vi "DS1000Z_Image_Grabber.vi"() -> ()   [LabVIEW 2020]
uses:
  <vilib>/Instr/_visa.llb/VISA Find Search Mode.ctl
  <vilib>/Utility/error.llb/DialogType.ctl
  <vilib>/Platform/browser.llb/Open URL in Default Browser (string).vi
  rigol_ds1000_series/RIGOL DS1000 Series/RIGOL DS1000 Series.lvlib
panel:
  in  "weblink":bool
  in  "Mode":u16(ring) items=["Single", "Stop"]
  in  "Set Trigger":bool
  in  "Trigger Delay":u32 format="%d sec"
  in  "Get Image":bool
  in  "Capture Delay":u32 format="%d sec"
  in  "File Name":string
  in  "Capture Storage Location":path
  in  "Invert":bool
  in  "Device Location":string(combo)
  in  "Format":u16(ring)=2 items=["24b BMP", "8b BMP", "PNG", "JPEG", "TIFF"]
  in  "Colour?":u16(ring) items=["Colour", "Grayscale"]
  # "Rigol DS1000Z-Series Oscilloscope PC Interface"
  # "© 2020 NixLabs  Version 0.56"
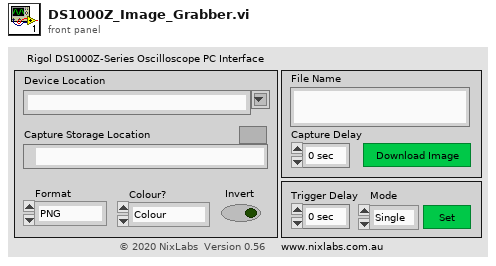
[diagram p1: front panel]
types:
  T1 = enum8{"Enabled", "Disabled", "Disabled and Grayed Out"}
  T2 = typedef "VISA Find Search Mode.ctl" = u32
  T3 = enum16{"big-endian, network order", "native, host order", "little-endian"}
  T4 = typedef "DialogType.ctl" = u16
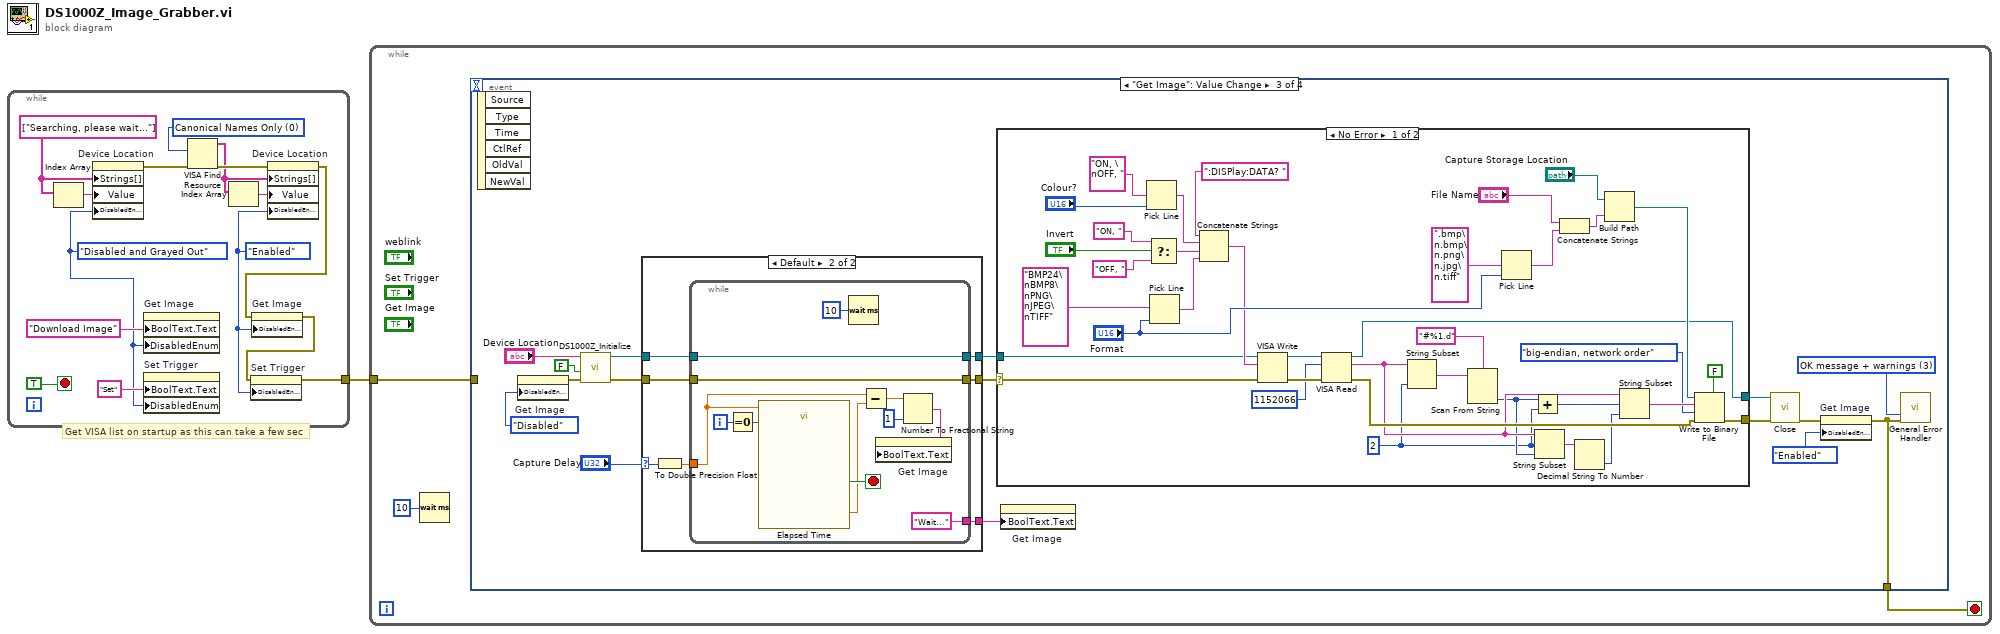
[diagram p0: block diagram]
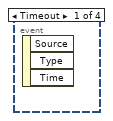
[diagram p2: hidden frame]
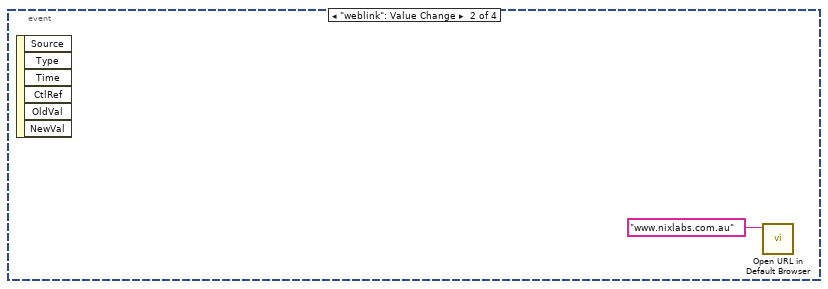
[diagram p3: hidden frame]
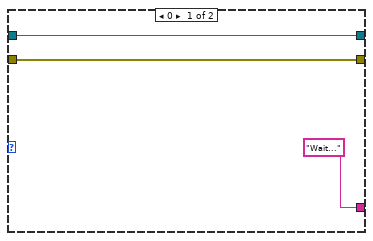
[diagram p4: hidden frame]
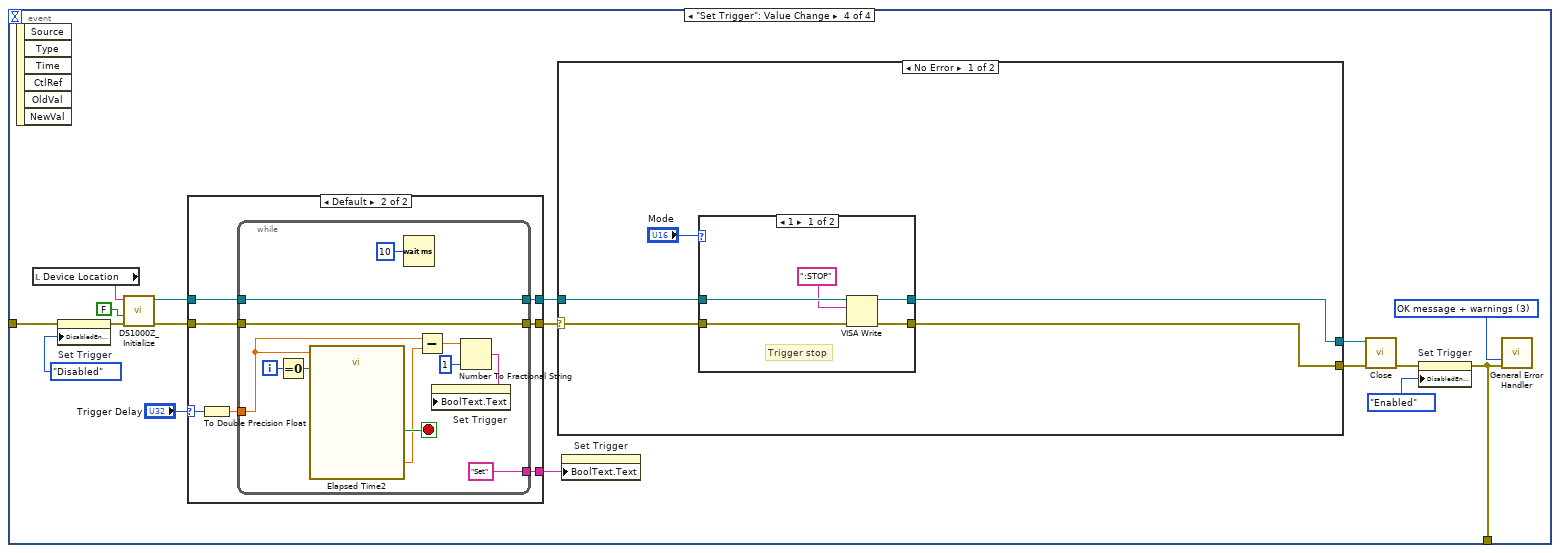
[diagram p6: hidden frame]
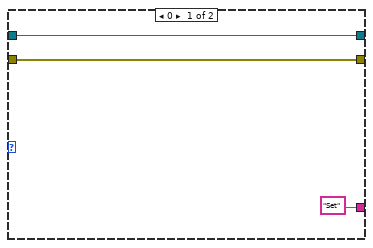
[diagram p7: hidden frame]
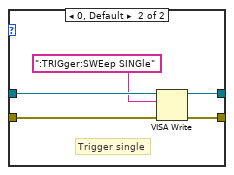
[diagram p8: hidden frame]
diagram:
  # "Get VISA list on startup as this can take a few sec"
  n1 = while {
    tunnel: [w2] -> w1
    stop <- TRUE stop-if-true
    w5 = T1."Enabled" ("Disabled")
    w6 = T1."Disabled and Grayed Out" ("Disabled")
    w10 = string[] ["Searching, please wait..."] ("array")
    w16 = T2 0 items=["Canonical Names Only"=0, "Aliases Only"=2, "Include Matching Aliases"=3, "Include All Aliases"=4] ("Search Mode")
    n2 = Index Array(array=w10) -> (element=w11:string)  [unwired: 1 in]
    n3 = property on="Device Location" class="CmbBox"("Strings[]"=w10, "Value"=w11, "DisabledEnum"=w6) -> (error out=w12:errorcluster)  [unwired: 2 in, 1 out]
    n4 = property on="Get Image" class="Bool"("BoolText.Text"="Download Image" ("Boolean Text.Text"), "DisabledEnum"=w6) -> ()  [unwired: 2 in, 2 out]
    n5 = property on="Set Trigger" class="Bool"("BoolText.Text"="Set" ("Boolean Text.Text"), "DisabledEnum"=w6) -> ()  [unwired: 2 in, 2 out]
    n6 = VISA Find Resource(8:w12, 10:w16) -> (0:w15:errorcluster, 3:w14:string[])  [unwired: 1 in, 1 out]
    n7 = Index Array(array=w14) -> (element=w13:string)  [unwired: 1 in]
    n8 = property on="Device Location" class="CmbBox"(error in=w15, "Strings[]"=w14, "Value"=w13, "DisabledEnum"=w5) -> (error out=w4:errorcluster)  [unwired: 1 in, 1 out]
    n9 = property on="Get Image" class="Bool"(error in=w4, "DisabledEnum"=w5) -> (error out=w3:errorcluster)  [unwired: 1 in, 1 out]
    n10 = property on="Set Trigger" class="Bool"(error in=w3, "DisabledEnum"=w5) -> (error out=w2:errorcluster)  [unwired: 1 in, 1 out]
  }
  n11 = while {
    tunnel: w1 -> [w17]
    stop <- w19 stop-if-true
    n12 = Wait (ms)(milliseconds to wait=u32 10) -> ()  [unwired: 1 out]
    n13 = event shown="[2] \"Get Image\": Value Change" {
      selector: _ -> [_ _ _ _]
      dyn-events: _ -> [_ _ _ _]
      timeout: _ -> [_ _ _ _]
      tunnel: [_ _ w22 w101] -> w19
      tunnel: w17 -> [_ _ _ w99]
      event Timeout {
        n14 = event-data() -> ()  [unwired: 1 in, 3 out]
      }
      event "weblink": Value Change {
        n15 = event-data() -> ()  [unwired: 1 in, 6 out]
        n16 = call-poly <vilib>:"Open URL in Default Browser.vi"("URL"="www.nixlabs.com.au") -> ()  [unwired: 5 in, 2 out]
      }
      event "Get Image": Value Change {
        w36 = T4 3 items=["no dialog", "OK message", "continue or stop message", "OK message + warnings", "continue/stop + warnings"] ("type of dialog (OK msg:1)")
        n17 = event-data() -> ()  [unwired: 1 in, 6 out]
        n18 = property on="Get Image" class="Bool"("DisabledEnum"=T1."Disabled" ("Disabled")) -> (error out=w25:errorcluster)  [unwired: 2 in, 1 out]
        n19 = call "DS1000Z_Initialize.vi"("error in (no error)"=w25, "Reset (True)"=FALSE, "VISA resource name"="Device Location") -> ("error out"=w30:errorcluster, "VISA resource name out"=w32:refnum<visa-resource-name>)  [unwired: 7 in]
        n20 = case shown="Default" "Capture Delay" {
          selector: "Capture Delay" -> [_ w41]
          tunnel: [w38 w46] -> w33
          tunnel: w32 -> [w38 w45]
          tunnel: [w39 w44] -> w31
          tunnel: w30 -> [w39 w43]
          tunnel: ["Wait..." w42] -> w29
          frame 0 {
          }
          frame Default {
            n21 = To Double Precision Float(number=w41) -> (double precision float=w40:dbl)
            n22 = while {
              tunnel: [w56] -> w46
              tunnel: w45 -> [w56]
              tunnel: [w55] -> w44
              tunnel: w43 -> [w55]
              tunnel: ["Wait..."] -> w42
              tunnel: w40 -> [w52]
              i -> [w48]
              stop <- w53 stop-if-true
              n23 = Equal To 0?(x=w48) -> (x = 0?=w47:bool)
              n24 = call "Elapsed Time"("Time Target (s)"=w52, "Reset"=w47) -> ("Elapsed Time (s)"=w51:dbl, "Time has Elapsed"=w53:bool)  [unwired: 10 in, 6 out]
              n25 = Wait (ms)(milliseconds to wait=u32 10) -> ()  [unwired: 1 out]
              n26 = Subtract(x=w52, y=w51) -> (x-y=w50:dbl)
              n27 = Number To Fractional String(number=w50, precision (6)=i16 1) -> (F-format string=w57:string)  [unwired: 2 in]
              n28 = property on="Get Image" class="Bool"("BoolText.Text"=w57) -> ()  [unwired: 2 in, 2 out]
            }
          }
        }
        n29 = case shown="No Error" w31 {
          selector: w31 -> [w60 w97]
          tunnel: [w95 w97] -> w35
          tunnel: w33 -> [w59 w96]
          tunnel: [w61 w96] -> w34
          frame No Error {
            w64 = 2 ("length (rest)")
            n30 = Pick Line(multi-line string="ON, \nOFF, ", line index="Colour?") -> (output string=w83:string)  [unwired: 1 in]
            n31 = Select(t="ON, " ("write buffer"), s="Invert", f="OFF, " ("write buffer")) -> (s? t:f=w84:string)
            n32 = Pick Line(multi-line string="BMP24\nBMP8\nPNG\nJPEG\nTIFF", line index="Format") -> (output string=w85:string)  [unwired: 1 in]
            n33 = Concatenate Strings(":DISPlay:DATA? " ("write buffer"), w83, w84, w85) -> (w86:string)
            n34 = VISA Write(VISA resource name=w59, write buffer=w86, error in (no error)=w60) -> (VISA resource name out=w74:refnum<visa-resource-name>, error out=w73:errorcluster)  [unwired: 1 out]
            n35 = VISA Read(VISA resource name=w74, byte count=u32 1152066, error in (no error)=w73) -> (VISA resource name out=w61:refnum<visa-resource-name>, read buffer=w81:string, error out=w82:errorcluster)  [unwired: 1 out]
            n36 = String Subset(string=w81, length (rest)=w64) -> (substring=w75:string)  [unwired: 1 in]
            n37 = Scan From String(format string="#%1.d", input string=w75) -> (output 1=w77:i32)  [unwired: 3 in, 3 out]
            n38 = Pick Line(multi-line string=".bmp\n.bmp\n.png\n.jpg\n.tiff", line index="Format") -> (output string=w89:string)  [unwired: 1 in]
            n39 = Add(x=w77, y=w64) -> (x+y=w79:i32)
            n40 = String Subset(string=w81, offset (0)=w64, length (rest)=w77) -> (substring=w76:string)
            n41 = Concatenate Strings("File Name", w89) -> (w88:string)
            n42 = Decimal String To Number(string=w76) -> (number=w78:i32)  [unwired: 2 in, 1 out]
            n43 = Build Path(base path="Capture Storage Location", name or relative path=w88) -> (appended path=w87:path)
            n44 = String Subset(string=w81, offset (0)=w79, length (rest)=w78) -> (substring=w80:string)
            n45 = Write to Binary File(file (use dialog)=w87, data=w80, error in=w82, 5:FALSE ("prepend array or string size? (T)"), 9:T3."big-endian, network order" ("byte order (0:big-endian, network order)")) -> (error out=w95:errorcluster)  [unwired: 1 in, 2 out]
          }
          frame Error {
          }
        }
        n46 = property on="Get Image" class="Bool"("BoolText.Text"=w29) -> ()  [unwired: 2 in, 2 out]
        n47 = call "Close.vi"("error in (no error)"=w35, "VISA resource name"=w34) -> ("error out"=w23:errorcluster)  [unwired: 9 in]
        n48 = property on="Get Image" class="Bool"(error in=w23, "DisabledEnum"=T1."Enabled" ("Disabled")) -> (error out=w22:errorcluster)  [unwired: 1 in, 1 out]
        n49 = call <vilib>:"General Error Handler.vi"("type of dialog (OK msg:1)"=w36, "error in (no error)"=w22) -> ()  [unwired: 9 in, 5 out]
      }
      event "Set Trigger": Value Change {
        w114 = T4 3 items=["no dialog", "OK message", "continue or stop message", "OK message + warnings", "continue/stop + warnings"] ("type of dialog (OK msg:1)")
        n50 = event-data() -> ()  [unwired: 1 in, 6 out]
        n51 = local read "Device Location"() -> (w98:string)
        n52 = property on="Set Trigger" class="Bool"(error in=w99, "DisabledEnum"=T1."Disabled" ("Disabled")) -> (error out=w104:errorcluster)  [unwired: 1 in, 1 out]
        n53 = call "DS1000Z_Initialize.vi"("error in (no error)"=w104, "Reset (True)"=FALSE, "VISA resource name"=w98) -> ("error out"=w108:errorcluster, "VISA resource name out"=w110:refnum<visa-resource-name>)  [unwired: 7 in]
        n54 = case shown="Default" "Trigger Delay" {
          selector: "Trigger Delay" -> [_ w119]
          tunnel: [w116 w124] -> w111
          tunnel: w110 -> [w116 w123]
          tunnel: [w117 w122] -> w109
          tunnel: w108 -> [w117 w121]
          tunnel: ["Set" w120] -> w107
          frame 0 {
          }
          frame Default {
            n55 = To Double Precision Float(number=w119) -> (double precision float=w118:dbl)
            n56 = while {
              tunnel: [w134] -> w124
              tunnel: w123 -> [w134]
              tunnel: [w133] -> w122
              tunnel: w121 -> [w133]
              tunnel: ["Set"] -> w120
              tunnel: w118 -> [w130]
              i -> [w126]
              stop <- w131 stop-if-true
              n57 = Equal To 0?(x=w126) -> (x = 0?=w125:bool)
              n58 = call "Elapsed Time2"("Time Target (s)"=w130, "Reset"=w125) -> ("Elapsed Time (s)"=w129:dbl, "Time has Elapsed"=w131:bool)  [unwired: 10 in, 6 out]
              n59 = Wait (ms)(milliseconds to wait=u32 10) -> ()  [unwired: 1 out]
              n60 = Subtract(x=w130, y=w129) -> (x-y=w128:dbl)
              n61 = Number To Fractional String(number=w128, precision (6)=i16 1) -> (F-format string=w135:string)  [unwired: 2 in]
              n62 = property on="Set Trigger" class="Bool"("BoolText.Text"=w135) -> ()  [unwired: 2 in, 2 out]
            }
          }
        }
        n63 = case shown="No Error" w109 {
          selector: w109 -> [w141 w153]
          tunnel: [w137 w153] -> w113
          tunnel: w111 -> [w140 w152]
          tunnel: [w139 w152] -> w112
          frame No Error {
            n64 = case shown="1" "Mode" {
              tunnel: w141 -> [w146 w151]
              tunnel: w140 -> [w145 w150]
              tunnel: [w143 w148] -> w139
              tunnel: [w142 w147] -> w137
              frame 1 {
                # "Trigger stop"
                n65 = VISA Write(VISA resource name=w145, write buffer=":STOP", error in (no error)=w146) -> (VISA resource name out=w143:refnum<visa-resource-name>, error out=w142:errorcluster)  [unwired: 1 out]
              }
              frame 0, Default {
                # "Trigger single"
                n66 = VISA Write(VISA resource name=w150, write buffer=":TRIGger:SWEep SINGle", error in (no error)=w151) -> (VISA resource name out=w148:refnum<visa-resource-name>, error out=w147:errorcluster)  [unwired: 1 out]
              }
            }
          }
          frame Error {
          }
        }
        n67 = property on="Set Trigger" class="Bool"("BoolText.Text"=w107) -> ()  [unwired: 2 in, 2 out]
        n68 = call "Close.vi"("error in (no error)"=w113, "VISA resource name"=w112) -> ("error out"=w102:errorcluster)  [unwired: 9 in]
        n69 = property on="Set Trigger" class="Bool"(error in=w102, "DisabledEnum"=T1."Enabled" ("Disabled")) -> (error out=w101:errorcluster)  [unwired: 1 in, 1 out]
        n70 = call <vilib>:"General Error Handler.vi"("type of dialog (OK msg:1)"=w114, "error in (no error)"=w101) -> ()  [unwired: 9 in, 5 out]
      }
    }
  }
